vi "Initialize UI.vi"(8 "error in (no error)":errorcluster) -> (0 "error out":errorcluster)   [LabVIEW 2019, in "GaitDAQ UI.lvlib"]
uses:
  GaitDAQ UI.lvlib
  <vilib>/Utility/sysdir.llb/System Directory Type.ctl
panel:
  # "Input"
  # "Output"
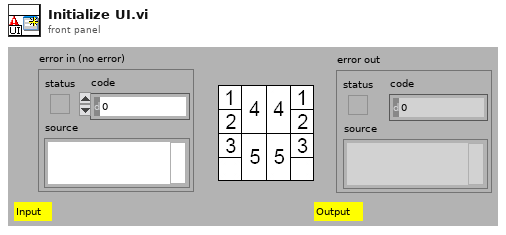
[diagram p1: front panel]
types:
  T1 = enum8{"Enabled", "Disabled", "Disabled and Grayed Out"}
  T2 = typedef "System Directory Type.ctl" = i32
  T3 = typedef "GaitDAQ UI.lvlib/UI Refnums.ctl" = cluster{"Exit Refnum":refnum<vi>, "Camera Open or Close":refnum<vi>, "Camera Discover":refnum<vi>, "Camera":refnum<vi>, "Log or Unlog":refnum<vi>, "COM Open or Close":refnum<vi>, "COM Port":refnum<vi>, "Play or Pause":refnum<vi>, "Foot Image":refnum<vi>, "Data Path 1":refnum<vi>, "Folder":refnum<vi>, "Data Path 2":refnum<vi>, "Acquire or Review":refnum<vi>, "Slide":refnum<vi>, "Load or Stop":refnum<vi>}
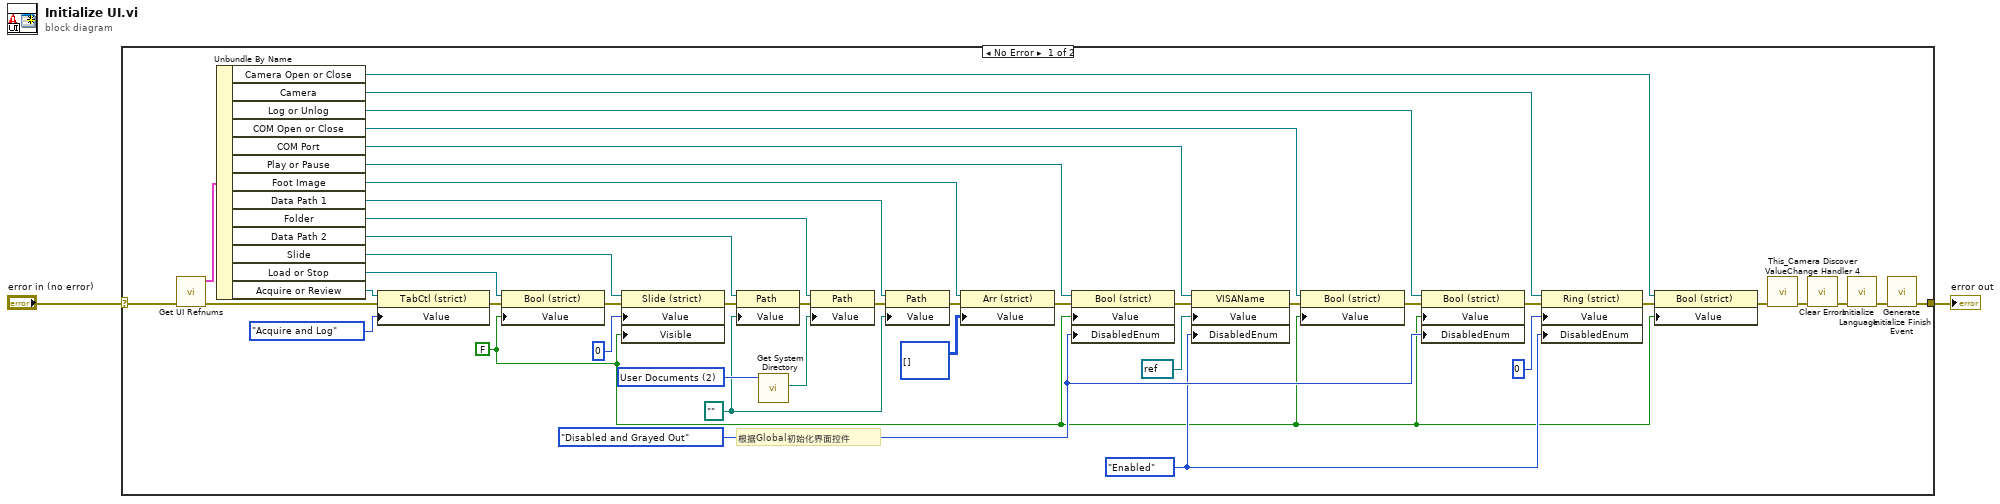
[diagram p0: block diagram]
diagram:
  n1 = case shown="No Error" "error in (no error)" {
    selector: "error in (no error)" -> [w44 w47]
    tunnel: [w45 w47] -> w1
    frame No Error {
      w7 = T1."Enabled" ("Disabled")
      w27 = path "" ("Value")
      w32 = T2 2 items=["User Home"=0, "User Desktop"=1, "User Documents"=2, "User Application Data"=3, "User Preferences"=4, "User Temporary"=5, "Public Documents"=6, "Public Application Data"=7, "Public Preferences"=8, "Public Cache"=13, "System Core Libraries"=9, "System Installed Libraries"=10, "Application Files"=11, "Boot Volume Root"=12] ("system directory type")
      w23 = T1."Disabled and Grayed Out" ("Disabled")
      w3 = FALSE ("Value")
      # "根据Global初始化界面控件"
      n2 = call "Get UI Refnums.vi"("error in (no error)"=w44) -> ("error out"=w20:errorcluster, "Button 0 Refnum Out"=w40:T3)  [unwired: 9 in]
      n3 = Unbundle By Name(w40) -> ("Camera Open or Close"=w43:refnum<vi>, "Camera"=w42:refnum<vi>, "Log or Unlog"=w39:refnum<vi>, "COM Open or Close"=w38:refnum<vi>, "COM Port"=w37:refnum<vi>, "Play or Pause"=w35:refnum<vi>, "Foot Image"=w34:refnum<vi>, "Data Path 1"=w29:refnum<vi>, "Folder"=w30:refnum<vi>, "Data Path 2"=w28:refnum<vi>, "Slide"=w26:refnum<vi>, "Load or Stop"=w24:refnum<vi>, "Acquire or Review"=w22:refnum<vi>)
      n4 = property class="TabCtl (strict)"(reference=w22, error in=w20, "Value"=enum32{"Acquire and Log", "Review"}."Acquire and Log") -> (error out=w19:errorcluster)  [unwired: 1 out]
      n5 = property class="Bool (strict)"(reference=w24, error in=w19, "Value"=w3) -> (error out=w18:errorcluster)  [unwired: 1 out]
      n6 = property class="Slide (strict)"(reference=w26, error in=w18, "Value"=u32 0, "Visible"=w3) -> (error out=w17:errorcluster)  [unwired: 1 out]
      n7 = property class="Path"(reference=w28, error in=w17, "Value"=w27) -> (error out=w16:errorcluster)  [unwired: 1 out]
      n8 = call <vilib>:"Get System Directory.vi"("system directory type"=w32) -> ("system directory"=w31:path)  [unwired: 10 in]
      n9 = property class="Path"(reference=w30, error in=w16, "Value"=w31) -> (error out=w15:errorcluster)  [unwired: 1 out]
      n10 = property class="Path"(reference=w29, error in=w15, "Value"=w27) -> (error out=w14:errorcluster)  [unwired: 1 out]
      n11 = property class="Arr (strict)"(reference=w34, error in=w14, "Value"=u32[][] []) -> (error out=w13:errorcluster)  [unwired: 1 out]
      n12 = property class="Bool (strict)"(reference=w35, error in=w13, "Value"=w3, "DisabledEnum"=w23) -> (error out=w8:errorcluster)  [unwired: 1 out]
      n13 = property class="VISAName"(reference=w37, error in=w8, "Value"=refnum<visa-resource-name> refnum, "DisabledEnum"=w7) -> (error out=w9:errorcluster)  [unwired: 1 out]
      n14 = property class="Bool (strict)"(reference=w38, error in=w9, "Value"=w3) -> (error out=w10:errorcluster)  [unwired: 1 out]
      n15 = property class="Bool (strict)"(reference=w39, error in=w10, "Value"=w3, "DisabledEnum"=w23) -> (error out=w11:errorcluster)  [unwired: 1 out]
      n16 = property class="Ring (strict)"(reference=w42, error in=w11, "Value"=u16 0, "DisabledEnum"=w7) -> (error out=w12:errorcluster)  [unwired: 1 out]
      n17 = property class="Bool (strict)"(reference=w43, error in=w12, "Value"=w3) -> (error out=w6:errorcluster)  [unwired: 1 out]
      n18 = call "This_Camera Discover ValueChange Handler 4.vi"("error in (no error)"=w6) -> ("error out"=w5:errorcluster)  [unwired: 10 in]
      n19 = call <vilib>:"Clear Errors.vi"("error in (no error)"=w5) -> ("error out"=w4:errorcluster)  [unwired: 5 in, 1 out]
      n20 = call "Initialize Language.vi"("error in (no error)"=w4) -> ("error out"=w46:errorcluster)  [unwired: 10 in]
      n21 = call "Generate Initialize Finish Event.vi"("error in (no error)"=w46) -> ("error out"=w45:errorcluster)  [unwired: 10 in]
    }
    frame Error {
    }
  }
  "error out" <- w1
